vi "Shut_down_all_Axis.vi"() -> (0 "Error String":string)   [LabVIEW 2022 SP3]
uses:
  DriveConfigGlobal.vi
  GenericDriveCommand.ctl
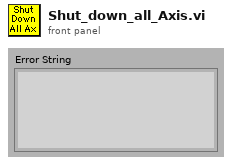
[diagram p1: front panel]
types:
  T1 = typedef "DriveProperties.ctl" = cluster{"Channel Name":string, "Vel. Default":sgl, "Acc. Default":sgl, "Vel. Max":sgl, "Vel. Min":sgl, "Acc. Max":sgl, "Acc. Min":sgl, "Pulses/unit":sgl, "Address":u8, "Pulse Offset":i32, "Pos Tolerance":sgl, "Pulses/rev":sgl, "Backlash/Eng units":sgl, "Current Pos":sgl, "Ch Status":enum16{"Active", "Offline", "Simulate"}, "Port Name":string, "Axis Transform mode":string, "Metadata Ch Name":string, "Type":string, "De Power Motor":enum16{"TRUE", "FALSE"}, "ConfigString":string}
  T2 = typedef "GenericDriveCommand.ctl" = string
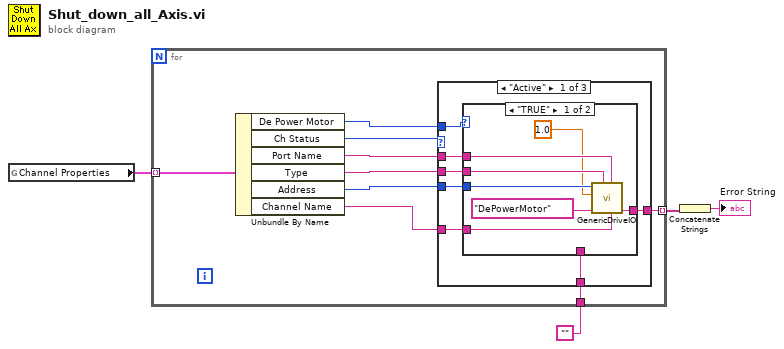
[diagram p0: block diagram]
diagram:
  n1 = global read "DriveConfigGlobal.vi" "Channel Properties"() -> (w4:T1[])
  n2 = for {
    tunnel: w4 -> [w13] mode=indexing
    tunnel: [w6] -> w3 mode=indexing
    tunnel: "" -> [w5]
    n3 = Unbundle By Name(w13) -> ("De Power Motor"=w7:enum16{"TRUE", "FALSE"}, "Ch Status"=w12:enum16{"Active", "Offline", "Simulate"}, "Port Name"=w11:string, "Type"=w10:string, "Address"=w9:u8, "Channel Name"=w8:string)
    n4 = case shown="\"Active\"" w12 {
      tunnel: w11 -> [w20 _ _]
      tunnel: w10 -> [w19 _ _]
      tunnel: w9 -> [w18 _ _]
      tunnel: w8 -> [w17 _ _]
      tunnel: w7 -> [w16 _ _]
      tunnel: [w15 w29 w30] -> w6
      tunnel: w5 -> [w14 w29 w30]
      frame "Active" {
        n5 = case shown="\"TRUE\"" w16 {
          tunnel: w20 -> [w27 _]
          tunnel: w19 -> [w26 _]
          tunnel: w18 -> [w25 _]
          tunnel: w17 -> [w24 _]
          tunnel: [w21 w28] -> w15
          tunnel: w14 -> [_ w28]
          frame "TRUE" {
            n6 = call "GenericDriveIO.vi"("GenericDriveCommand"=T2 "DePowerMotor", "Channel Name"=w24, "Numeric Value"=1.0, "Address"=w25, "Type"=w26, "Port Name"=w27) -> ("Error Description"=w21:string)  [unwired: 1 in, 4 out]
          }
          frame "FALSE" {
          }
        }
      }
      frame "Offline" {
      }
      frame "Simulate" {
      }
    }
  }
  n7 = Concatenate Strings(w3) -> (→"Error String":string)
